vi "写测试报告到标准库.vi"(6 "delimiter (\\t)":string=",", 9 "1D data":string[](array[string]) caption="一维数据", 10 "表头":string[][](array[string]), 11 "写入配置文件地址":path caption="文件路径 （空时为对话框）") -> ()   [LabVIEW 2016]
uses:
  <vilib>/Utility/file.llb/Write Delimited Spreadsheet (string).vi
panel:
  in  "format (%s)":string="%s" caption="格式(%.3f)"
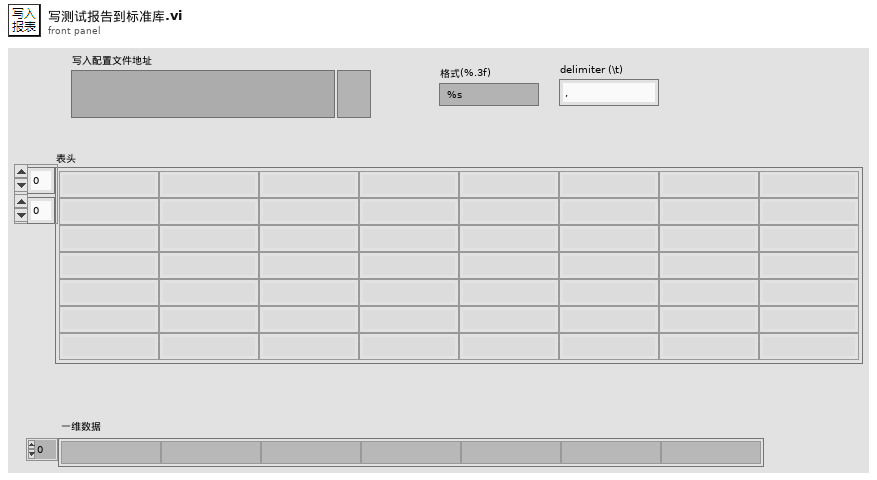
[diagram p1: front panel]
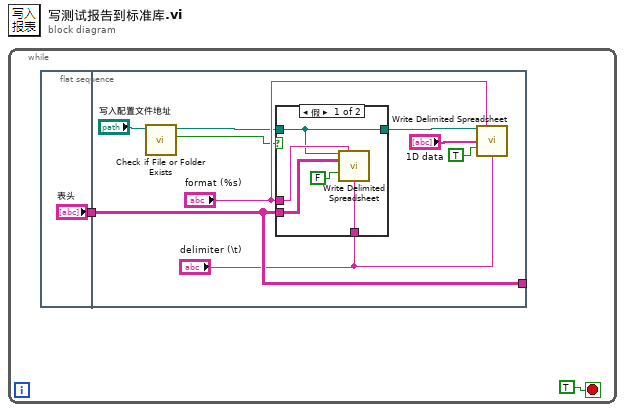
[diagram p0: block diagram]
diagram:
  n1 = while {
    stop <- TRUE stop-if-true
    n2 = flat-sequence {
      tunnel: ["表头"] -> w1
      tunnel: w1 -> [w10]
      tunnel: [w10] -> _
      frame #0 {
      }
      frame #1 {
        n3 = call <vilib>:"Check if File or Folder Exists.vi"("path"="写入配置文件地址") -> ("file or folder exists?"=w8:bool, "dup path"=w7:path)  [unwired: 8 in, 1 out]
        n4 = case shown="假" w8 {
          tunnel: w7 -> [w15 w18]
          tunnel: "format (%s)" -> [w16 _]
          tunnel: w10 -> [w14 _]
          tunnel: [w15 w18] -> w6
          tunnel: "delimiter (\\t)" -> [w13 _]
          frame False {
            n5 = call-poly <vilib>:"Write Delimited Spreadsheet.vi"("file path (dialog if empty)"=w15, "format (%s)"=w16, "2D data"=w14, "append to file? (new file:F)"=FALSE, "delimiter (\\t)"=w13) -> ()  [unwired: 9 in, 2 out]
          }
          frame True {
          }
        }
        n6 = call-poly <vilib>:"Write Delimited Spreadsheet.vi"("file path (dialog if empty)"=w6, "format (%s)"="format (%s)", "1D data"="1D data", "append to file? (new file:F)"=TRUE, "delimiter (\\t)"="delimiter (\\t)") -> ()  [unwired: 9 in, 2 out]
      }
    }
  }
